vi "Configure.vi"(8 "error in (no error)":errorcluster, 11 "IMAQ Camera in":refnum<class "IMAQ Camera.lvclass">) -> (0 "error out":errorcluster, 3 "IMAQ Camera out":refnum<class "IMAQ Camera.lvclass">)   [LabVIEW 2011, in "IMAQ Camera.lvclass"]
uses:
  IMAQ Camera.lvclass
  IMAQ Camera.lvclass/IMAQ Camera.ctl
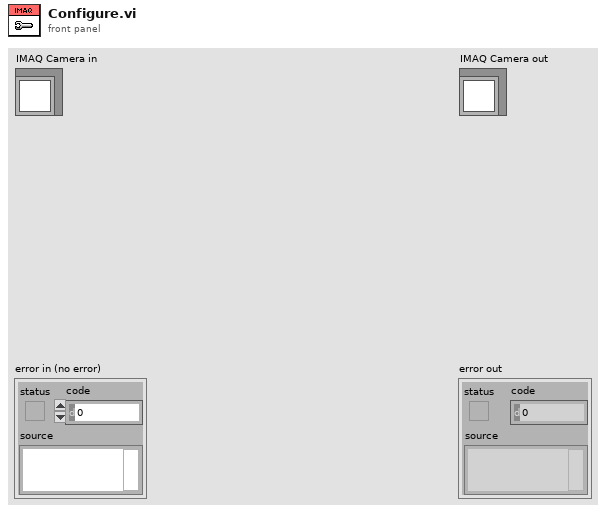
[diagram p1: front panel]
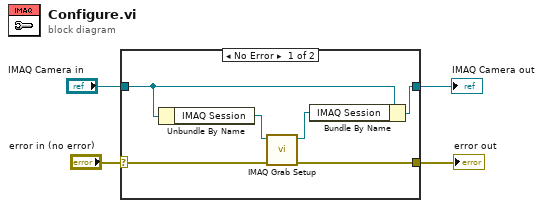
[diagram p0: block diagram]
diagram:
  n1 = case shown="No Error" "error in (no error)" {
    selector: "error in (no error)" -> [w5 w11]
    tunnel: "IMAQ Camera in" -> [w9 w12]
    tunnel: [w7 w12] -> w3
    tunnel: [w6 w11] -> w2
    frame No Error {
      n2 = Unbundle By Name(w9) -> ("IMAQ Session"=w10:refnum<k11>)
      n3 = call <vilib>:"IMAQ Grab Setup.vi"("error in (no error)"=w5, "IMAQ Session In"=w10) -> ("error out"=w6:errorcluster, "IMAQ Session Out"=w8:refnum<k11>)  [unwired: 8 in]
      n4 = Bundle By Name(cluster=w9, "IMAQ Session"=w8) -> (w7:refnum<class "IMAQ Camera.lvclass">)
    }
    frame Error {
    }
  }
  "error out" <- w2
  "IMAQ Camera out" <- w3
